vi "Image_Save_Handler.vi"(0 "first iteration":bool, 4 "Data":T3={"Pinch-valve"="Test Sample", "XLP 6000 Pump"="MRJ", "Camera1"="", "Camera2"="", "Img_Capt"=FALSE, "Actuator"=FALSE, "Pump"=FALSE, "Cam 1"=FALSE, "Cam 2"=FALSE, "Empty_Refill"=FALSE, "Crop"=FALSE, "Light intensity"=0, "Exposure Time"=0.0, "Sample Name"="", "Operator"="", "Calibration 1"=path "C:/Users/au540322/Desktop/IHS_Project/images/Debris/Debris_0/Debris_0_2019_06_01-23-32-49-686.PNG", "Calibration 2"=path "C:/Users/au540322/Desktop/IHS_Project/images/Debris/Debris_0/Debris_0_2019_06_01-23-32-49-686.PNG", "Framerate"=1, "Timeout Sample"=1, "Collection date"="", "Sample size threshold"=500, "Empty start"=500, "Command"="", "Station"="", "Species Name"="", "Other Notes"="", "Aperture"=enum."Item 3", "Image Process Queue Size"=100, "Image Save Queue Size"=0, "Overload threshold"=0, "Max Framerate"=0, "Rectangle 1"={"Left"=0, "Top"=0, "Right"=0, "Bottom"=0, "Rotation"=0.0}, "Rectangle 2"={"Left"=0, "Top"=100, "Right"=100, "Bottom"=0, "Rotation"=0.0}, "Detection Region %"=200.0, "Detect 1"=path "C:/Users/au540322/Desktop/IHS_Project/images/Debris/Debris_0/Debris_0_2019_06_01-23-32-49-686.PNG", "Detect 2"=path "C:/Users/au540322/Desktop/IHS_Project/images/Debris/Debris_0/Debris_0_2019_06_01-23-32-49-686.PNG", "Max large object threshold"=500, "Open(T)/Close(F)"=FALSE, "Img_Capt Begin"=FALSE, "Dispense Speed"=0, "Flush Size"=0, "Location"="", "Latitude"="", "Longitude"="", "Determiner"="", "Sex"="", "Camera1_Img"=refnum, "Camera2_Img"=refnum, "Img1_Orig_Disp"=refnum, "Img2_Orig_Disp"=refnum, "Img1_Orig_RGB"=refnum, "Img2_Orig_RGB"=refnum, "Blue_Plane_Extract"=refnum, "Subtracted_Plane"=refnum, "Img1_Binary"=refnum, "Img2_Binary"=refnum, "Crop_Mask"=refnum, "Img1_Save"=refnum, "Img2_Save"=refnum, "Img1_Cali_Full"=refnum, "Img2_Cali_Full"=refnum, "Img1_Cali_Detect"=refnum, "Img2_Cali_Detect"=refnum, "Cam 1 queue"=refnum, "Cam 2 queue"=refnum, "Cam 1 - save queue"=refnum, "Cam 2 - save queue"=refnum, "Overlay_Ring"=0, "SystemVersion"=0, "System Serial"="", "Legacy Cam Attributes"=FALSE, "Camera Orientation 1"="", "Camera Orientation 2"="", "Pixel to mm 1"=0.0, "Pixel to mm 2"=0.0, "CAM1 Model"=enum."a2A5328-15ucBAS", "CAM2 Model"=enum."a2A5328-15ucBAS", "Flush Insect"=FALSE, "Pump Size"=FALSE, "Barcode"="", "Phase3"=FALSE, "Mega F3"="", "Container nr."=0.0, "Flush Error"=TRUE, "Start System"=FALSE, "Size Interval"=0.0, "Mun. of containers"=0.0, "Sorting sys."=FALSE, "Initial size"=0.0} {"SystemVersion" items=["Standard", "XL"]; "Overlay_Ring" items=["Session Data", "Extended Setup", "Buffer", "Camera", "Dispenser", "Stats", "Connections"]; "Flush Size" min=1; "Dispense Speed" min=1; "Rectangle 2"."Rotation" format="%.2f"; "Rectangle 2"."Left" scale=0.0..1024.0; "Rectangle 2"."Right" scale=0.0..1024.0; "Rectangle 1"."Rotation" format="%.2f"; "Rectangle 1"."Left" scale=0.0..1024.0; "Rectangle 1"."Right" scale=0.0..1024.0; "Max Framerate" min=1; "Overload threshold" min=1; "Image Save Queue Size" min=1; "Image Process Queue Size" min=1; "Empty start" min=1; "Sample size threshold" min=1; "Framerate" min=1; "Light intensity" scale=0.0..100.0}, 7 "Stop?":bool) -> (12 "Image Save 1":T1, 14 "Image Save 2":T1, 15 "Container barcode":string, 17 "Cam2_Stats":cluster{"Mean_Area":i32, "Img_Count":u32} caption="Camera 2", 18 "Ready file created":bool, 19 "Cam1_Stats":cluster{"Mean_Area":i32, "Img_Count":u32} caption="Camera 1", 20 "Queue size":T2, 23 "timeout":bool, 24 "max queue":i32, 25 "Sample Name":string, 27 "Stop out":bool)   [LabVIEW 2024]
doc: "Saves image files from cameras in specified folder location."
uses:
  controls/Data.ctl
  <vilib>/userDefined/High Color/IMAQdx.ctl
  <vilib>/vision/Image Controls.llb/IMAQ Image.ctl
  Camera_ID.ctl
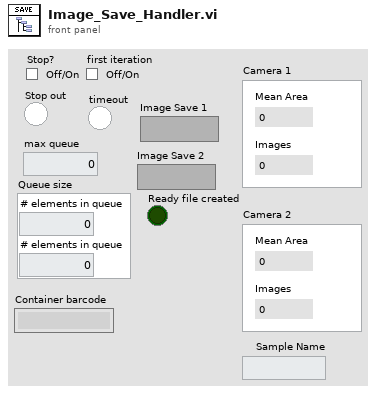
[diagram p1: front panel]
types:
  T1 = typedef "IMAQ Image.ctl" = refnum<image>
  T2 = cluster{"# elements in queue":i32, "# elements in queue":i32}
  T3 = typedef "Data.ctl" = cluster{"Pinch-valve":refnum<visa-resource-name>, "XLP 6000 Pump":refnum<visa-resource-name>, "Camera1":T4, "Camera2":T4, "Img_Capt":bool, "Actuator":bool, "Pump":bool, "Cam 1":bool, "Cam 2":bool, "Empty_Refill":bool, "Crop":bool, "Light intensity":i32, "Exposure Time":dbl, "Sample Name":string, "Operator":string, "Calibration 1":path, "Calibration 2":path, "Framerate":i32, "Timeout Sample":i32, "Collection date":string, "Sample size threshold":i32, "Empty start":u32, "Command":string, "Station":string, "Species Name":string, "Other Notes":string, "Aperture":enum32{"Item 0", "Item 1", "Item 2", "Item 3"}, "Image Process Queue Size":i32, "Image Save Queue Size":i32, "Overload threshold":i32, "Max Framerate":i32, "Rectangle 1":T5, "Rectangle 2":T5, "Detection Region %":dbl, "Detect 1":path, "Detect 2":path, "Max large object threshold":i32, "Open(T)/Close(F)":bool, "Img_Capt Begin":bool, "Dispense Speed":i32, "Flush Size":i32, "Location":string, "Latitude":string, "Longitude":string, "Determiner":string, "Sex":string, "Camera1_Img":T1, "Camera2_Img":T1, "Img1_Orig_Disp":T1, "Img2_Orig_Disp":T1, "Img1_Orig_RGB":T1, "Img2_Orig_RGB":T1, "Blue_Plane_Extract":T1, "Subtracted_Plane":T1, "Img1_Binary":T1, "Img2_Binary":T1, "Crop_Mask":T1, "Img1_Save":T1, "Img2_Save":T1, "Img1_Cali_Full":T1, "Img2_Cali_Full":T1, "Img1_Cali_Detect":T1, "Img2_Cali_Detect":T1, "Cam 1 queue":refnum<queue>, "Cam 2 queue":refnum<queue>, "Cam 1 - save queue":refnum<queue>, "Cam 2 - save queue":refnum<queue>, "Overlay_Ring":u16, "SystemVersion":u16, "System Serial":string, "Legacy Cam Attributes":bool, "Camera Orientation 1":string, "Camera Orientation 2":string, "Pixel to mm 1":dbl, "Pixel to mm 2":dbl, "CAM1 Model":enum16{"a2A5328-15ucBAS", "acA1920-155uc"}, "CAM2 Model":enum16{"a2A5328-15ucBAS", "acA1920-155uc"}, "Flush Insect":bool, "Pump Size":bool, "Barcode":string, "Phase3":bool, "Mega F3":refnum<visa-resource-name>, "Container nr.":dbl, "Flush Error":bool, "Start System":bool, "Size Interval":dbl, "Mun. of containers":dbl, "Sorting sys.":bool, "Initial size":dbl}
  T4 = typedef "IMAQdx.ctl" = refnum<k21>
  T5 = typedef "IMAQ Rectangle" = cluster{"Left":i32, "Top":i32, "Right":i32, "Bottom":i32, "Rotation":dbl}
  T6 = typedef "Camera_ID.ctl" = enum16{"Camera 1", "Camera 2"}
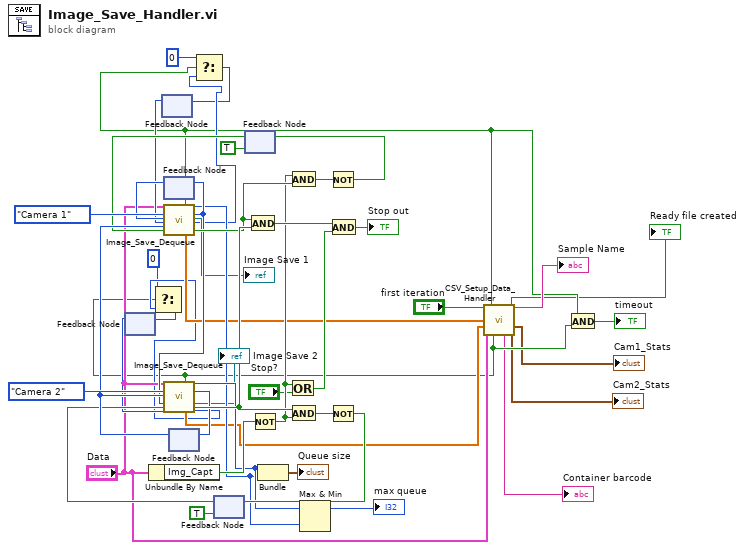
[diagram p0: block diagram]
diagram:
  n1 = feedback #1() -> (w14:u32)  [unwired: 1 in]
  n2 = Unbundle By Name("Data") -> ("Img_Capt"=w43:bool)
  n3 = feedback #2() -> (w15:u32)  [unwired: 1 in]
  n4 = feedback #3() -> (w36:i32)  [unwired: 1 in]
  n5 = feedback #4() -> (w34:i32)  [unwired: 1 in]
  n6 = feedback #5(TRUE) -> (w29:bool)
  n7 = feedback #6(TRUE) -> (w31:bool)
  n8 = call "Image_Save_Dequeue.vi"("Data"="Data", "Camera"=Camera_ID."Camera 1", "Old"=w36, "cam1_prev"=w15, "Other"=w34, "Queue active"=w31) -> ("timed out?"=w6:bool, "Sample Data"=w16:dbl[], "# elements in queue"=w24:i32, "State out"=w33:i32, "Image Save 1"=→"Image Save 1":T1, "cam1_count"=w12:u32, "Last image"=w40:bool)  [unwired: 13 in, 2 out]
  n9 = feedback-in #3(w33) -> ()
  n10 = call "Image_Save_Dequeue.vi"("Data"="Data", "Camera"=Camera_ID."Camera 2", "Old"=w34, "Other"=w33, "Queue active"=w29, "cam2_prev"=w14) -> ("timed out?"=w5:bool, "Sample Data"=w22:dbl[], "# elements in queue"=w25:i32, "State out"=w35:i32, "Image Save 2"=→"Image Save 2":T1, "Last image"=w42:bool, "cam2_count"=w8:u32)  [unwired: 13 in, 2 out]
  n11 = Select(t=u32 0, s=w5, f=w8) -> (s? t:f=w9:u32)
  n12 = feedback-in #1(w9) -> ()
  n13 = feedback-in #4(w35) -> ()
  n14 = Select(t=u32 0, s=w6, f=w12) -> (s? t:f=w11:u32)
  n15 = feedback-in #2(w11) -> ()
  n16 = And(x=w40, y=w42) -> (x .and. y?=w46:bool)
  n17 = Not(x=w43) -> (.not. x?=w39:bool)
  n18 = Bundle("# elements in queue"=w25, "# elements in queue"=w24) -> (→"Queue size":T2)  [unwired: 1 in]
  n19 = Or(x=w39, y="Stop?") -> (x .or. y?=w44:bool)
  n20 = And(x=w39, y=w40) -> (x .and. y?=w38:bool)
  n21 = And(x=w42, y=w39) -> (x .and. y?=w41:bool)
  n22 = Max & Min(x=w25, y=w24) -> (max(x,y)=→"max queue":i32)  [unwired: 1 out]
  n23 = Not(x=w38) -> (.not. x?=w32:bool)
  n24 = feedback-in #6(w32) -> ()
  n25 = Not(x=w41) -> (.not. x?=w30:bool)
  n26 = feedback-in #5(w30) -> ()
  n27 = And(x=w46, y=w44) -> (x .and. y?=→"Stop out":bool)
  n28 = call "CSV_Setup_Data_Handler.vi"("first iteration"="first iteration", "Timeout 1"=w6, "Sample Data"=w16, "Sample Data 2"=w22, "Data"="Data", "Timeout 2"=w5) -> ("Sample Name"=→"Sample Name":string, "Ready file created"=→"Ready file created":bool, "Cam1_Stats"=→"Cam1_Stats":cluster{"Mean_Area":i32, "Img_Count":u32}, "Container barcode"=→"Container barcode":string, "Cam2_Stats"=→"Cam2_Stats":cluster{"Mean_Area":i32, "Img_Count":u32})  [unwired: 5 in]
  n29 = And(x=w6, y=w5) -> (x .and. y?=→"timeout":bool)
